vi "stop.vi"(8 "error in (no error)":errorcluster, 11 "CameraControlViewer in":refnum<class "CameraControlViewer.lvclass">) -> (0 "error out":errorcluster, 3 "CameraControlViewer out":refnum<class "CameraControlViewer.lvclass">)   [LabVIEW 2009, in "Views.lvlib" / "Camera.lvlib" / "CameraControlViewer.lvclass"]
uses:
  CameraControlViewer.lvclass
  CameraControlViewer.lvclass/CameraControlViewer.ctl
  Hal/HWController/HWControllerEvents/HWControllerEvents.lvclass
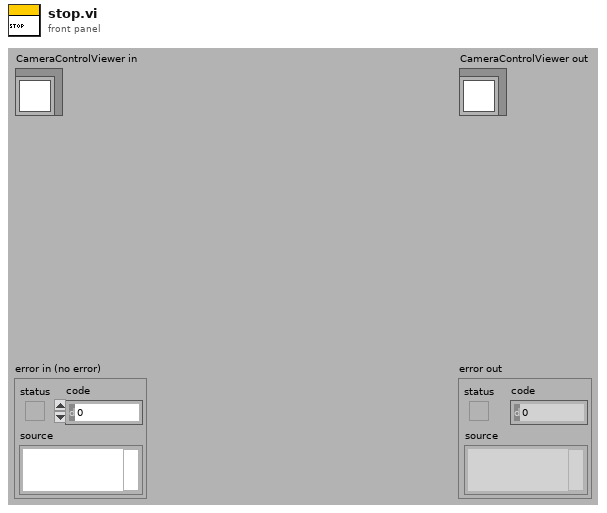
[diagram p1: front panel]
types:
  T1 = enum16{"start", "stop", "statusInquiry", "configure", "resetError", "resourcesInquiry", "reserveResources", "initialise", "resetAllChannels", "staticUpdate", "close", "HWStatus", "error", "resourcesAvailable", "resourcesReserved", "compilerError", "compiledScript", "compilingScript", "runScript", "configureCompiledScript", "restartCompiler", "staticRfChannelUpdate", "cameraUpdate"}
  T2 = cluster{"incomingEventTypes":cluster{"start":cluster{"Boolean":bool}, "stop":cluster{"Boolean":bool}, "statusInquiry":cluster{"Boolean":bool}, "configure":cluster{"DPScriptPath":path, "TimeStamp":string, "HWLoop?":bool}, "resetError":cluster{"Boolean":bool}, "resourcesInquiry":cluster{"Boolean":bool}, "reserveResources":cluster{"HWList":string[]}, "initialise":cluster{"HWList":string[]}, "close":cluster{"Boolean":bool}, "resetAllChannels":cluster{"Boolean":bool}, "staticChannelUpdate":cluster{"channel_address":string, "calibratedValue":dbl}, "runScript":cluster{"DPScriptPath":path, "TimeStamp":string, "HWLoop?":bool}, "compilingScript":cluster{"Path":path}, "compiledScript":cluster{"Path":path, "timeCompileAt":string}, "compilerError":cluster{"Path":path}, "configureCompiledScript":cluster{"DPScriptPath":path, "TimeStamp":string, "HWLoop?":bool, "CompiledScript":cluster{"ScriptListCompiler.lvclass":refnum<class "ScriptListCompiler.lvclass">, "aoChannels":refnum<class "AnalogOutput.lvclass">[], "doChannels":refnum<class "DigitalOutput.lvclass">[], "rfChannels":refnum<class "DDSOutput.lvclass">[]}}, "restartCompiler":cluster{"restart":bool}, "staticRfChannelUpdate":cluster{"channel_address":string, "Output":cluster{"Frequency(MHz)":dbl, "Amplitude":dbl, "Phase":dbl, "OutputForm":enum16{"Sine", "Square", "Triangle", "Arbitrary"}}}, "cameraUpdate":cluster{"Camera":string, "Type":string, "settings":path}}, "outgoingEventTypes":cluster{"HWStatus":cluster{"status":enum16{"Ready", "Compiling", "Configured", "Running", "Stopping", "Unresolved Error"}}, "error":cluster{"error out":errorcluster}, "resourcesAvailable":cluster{"availableHWList":string[], "reservedHWList":string[]}, "resourcesReserved":cluster{"reservedHWList":string[]}}}
  T3 = cluster{"Camera":string, "Type":string, "settings":path}
  T4 = cluster{"eventId":enum16{"start", "stop", "statusInquiry", "configure", "resetError", "resourcesInquiry", "reserveResources", "initialise", "resetAllChannels", "staticUpdate", "close", "HWStatus", "error", "resourcesAvailable", "resourcesReserved", "compilerError", "compiledScript", "compilingScript", "runScript", "configureCompiledScript", "restartCompiler", "staticRfChannelUpdate", "cameraUpdate"}, "cameraUpdate":cluster{"Camera":string, "Type":string, "settings":path}}
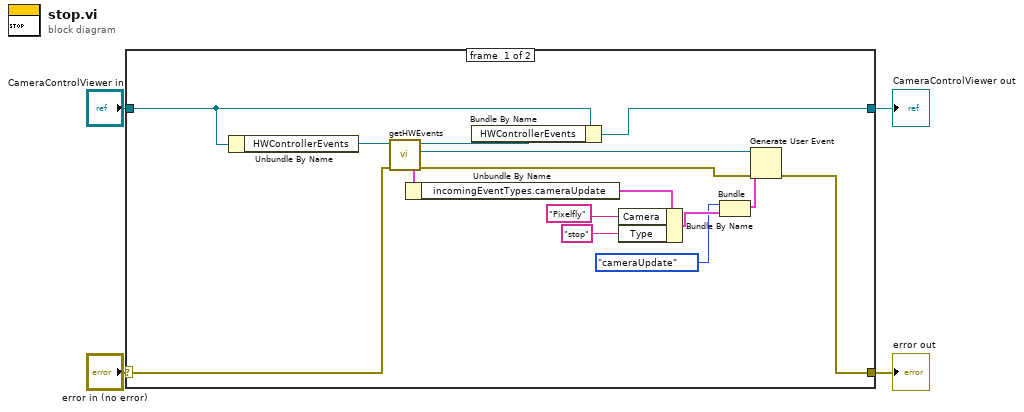
[diagram p0: block diagram]
diagram:
  n1 = case shown="No Error" "error in (no error)" {
    selector: "error in (no error)" -> [w7 w21]
    tunnel: [w6 w21] -> w3
    tunnel: [w8 w20] -> w1
    tunnel: "CameraControlViewer in" -> [w5 w20]
    frame #0 {
      n2 = Unbundle By Name(w5) -> ("HWControllerEvents"=w19:refnum<class "HWControllerEvents.lvclass">)
      n3 = call-dynamic "getHWEvents.vi"("error in (no error)"=w7, "HWControllerEvents in"=w19) -> ("error out"=w13:errorcluster, "eventDataTypes"=w18:T2, "HWCEvent"=w14:refnum<user-event>, "HWControllerEvents out"=w9:refnum<class "HWControllerEvents.lvclass">)  [unwired: 6 in]
      n4 = Unbundle By Name(w18) -> ("incomingEventTypes.cameraUpdate"=w17:T3)
      n5 = Bundle By Name(cluster=w5, "HWControllerEvents"=w9) -> (w8:refnum<class "CameraControlViewer.lvclass">)
      n6 = Bundle By Name(cluster=w17, "Camera"="Pixelfly", "Type"="stop") -> (w12:T3)
      n7 = Bundle("eventId"=T1."cameraUpdate", "cameraUpdate"=w12) -> (w10:T4)  [unwired: 1 in]
      n8 = Generate User Event(user event=w14, event data cluster=w10, error in=w13) -> (error out=w6:errorcluster)  [unwired: 1 out]
    }
    frame #1 {
    }
  }
  "error out" <- w3
  "CameraControlViewer out" <- w1
